vi "Set Iteration.vi"(7 "Progress Max":i32, 8 "error in (no error)":errorcluster {"code" format="Error %.0f"}, 9 "Progress Value":i32, 10 "Message (No Message Update)":string, 11 "UI Interaction in":refnum<class "UI Interaction.lvclass">) -> (0 "error out":errorcluster {"code" format="Error %.0f"}, 2 "Abort?":bool, 3 "UI Interaction out":refnum<class "UI Interaction.lvclass">)   [LabVIEW 2023, in "UI Interaction.lvclass"]
doc: "Wrapper that combines setting the Progress Max, Progress Value, and optionally the Message.\nReturns a check on Abort."
uses:
  UI Interaction.lvclass
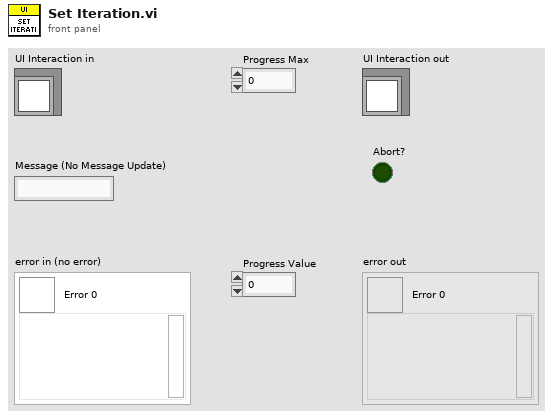
[diagram p1: front panel]
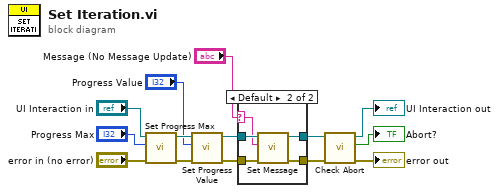
[diagram p0: block diagram]
diagram:
  n1 = call-dynamic "Set Progress Max.vi"("error in (no error)"="error in (no error)", "Progress Max"="Progress Max", "UI Interaction in"="UI Interaction in") -> ("error out"=w11:errorcluster, "UI Interaction out"=w14:refnum<class "UI Interaction.lvclass">)  [unwired: 7 in]
  n2 = call-dynamic "Set Progress Value.vi"("error in (no error)"=w11, "Progress Value"="Progress Value", "UI Interaction in"=w14) -> ("error out"=w10:errorcluster, "UI Interaction out"=w13:refnum<class "UI Interaction.lvclass">)  [unwired: 7 in]
  n3 = case shown="Default" "Message (No Message Update)" {
    selector: "Message (No Message Update)" -> [_ w17]
    tunnel: w13 -> [w15 w21]
    tunnel: [w15 w20] -> w5
    tunnel: w10 -> [w16 w19]
    tunnel: [w16 w18] -> w3
    frame "" {
    }
    frame Default {
      n4 = call-dynamic "Set Message.vi"("error in (no error)"=w19, "Message"=w17, "UI Interaction in"=w21) -> ("error out"=w18:errorcluster, "UI Interaction out"=w20:refnum<class "UI Interaction.lvclass">)  [unwired: 7 in]
    }
  }
  n5 = call-dynamic "Check Abort.vi"("error in (no error)"=w3, "UI Interaction in"=w5) -> ("error out"=→"error out":errorcluster, "Abort?"=→"Abort?":bool, "UI Interaction out"=→"UI Interaction out":refnum<class "UI Interaction.lvclass">)  [unwired: 7 in]
